vi "main.vi"   [LabVIEW 2020, in "GPackTools.lvlib" / "GPackAskPass.lvclass"]
uses:
  GPackAskPass.lvclass
  <vilib>/Wiresmith Technology/G CLI/CLI Class/CLI.lvclass
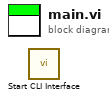
[diagram p0: block diagram]
diagram:
  n1 = call <vilib>:"Start CLI Interface.vi"() -> ()  [unwired: 8 in, 4 out]
